vi "Filelist.get.vi"(8 "error in (no error)":errorcluster, 11 "comic_crawler in":refnum<class "comic_crawler.lvclass">) -> (0 "error out":errorcluster, 2 "out of date filelist":path[](array[path]), 3 "comic_crawler out":refnum<class "comic_crawler.lvclass">)   [LabVIEW 2024, in "comic_crawler.lvclass"]
uses:
  comic_crawler.lvclass
  comic_crawler.lvclass/comic_crawler.ctl
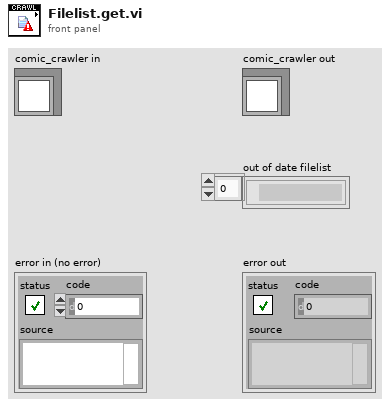
[diagram p1: front panel]
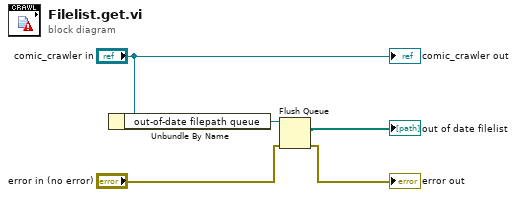
[diagram p0: block diagram]
diagram:
  n1 = Unbundle By Name("comic_crawler in") -> ("out-of-date filepath queue"=w4:refnum<queue>)
  n2 = Flush Queue(queue=w4, error in (no error)="error in (no error)") -> (remaining elements=→"out of date filelist":path[], error out=→"error out":errorcluster)  [unwired: 1 out]
  "comic_crawler out" <- "comic_crawler in"
